vi "Problem1.9-ExecutionTime.vi"() -> ()   [LabVIEW 2019]
panel:
  out "Execution Time (ms)":dbl
  out "Min Index":i32[](array[numeric])
  out "Max Index":i32[](array[numeric])
  out "Min Value":dbl
  out "Max Value":dbl
  out "Array Size":i32[](array[numeric])
  out "Original Random Number Array":dbl[][](array[numeric])
  out "Uniform Deviates Array":dbl[][](array[numeric])
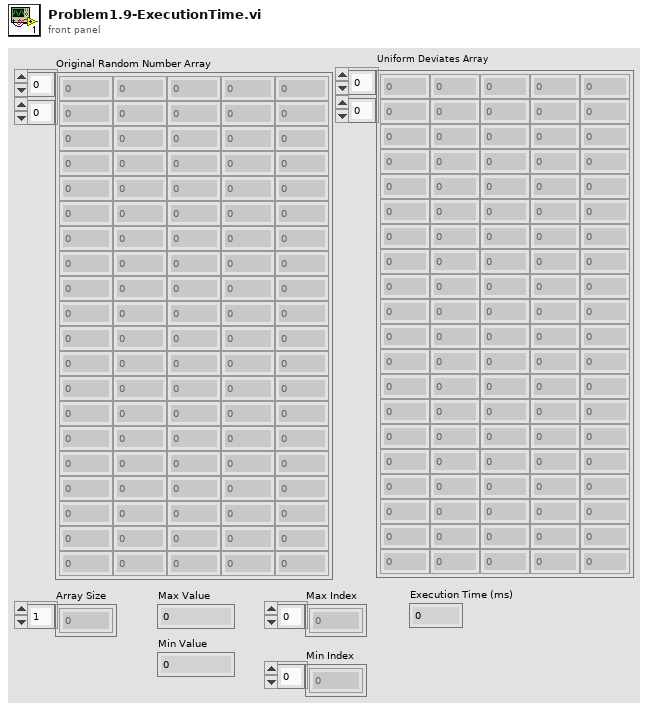
[diagram p1: front panel]
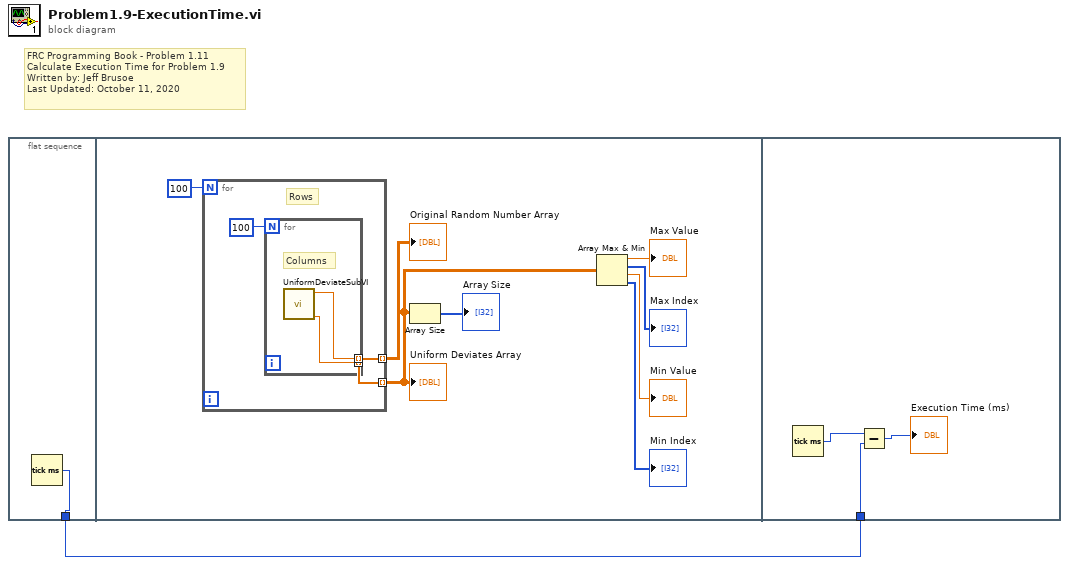
[diagram p0: block diagram]
diagram:
  # "FRC Programming Book - Problem 1.11\nCalculate Execution Time for Problem 1.9\nWritten by: Jeff Brusoe\nLast Updated: October 11, 2020"
  n1 = flat-sequence {
    tunnel: [w2] -> w1
    tunnel: w1 -> [w16]
    frame #0 {
      n2 = Tick Count (ms)() -> (millisecond timer value=w2:u32)
    }
    frame #1 {
      n3 = for {
        N: 100 -> [_]
        tunnel: [w12] -> w7 mode=indexing
        tunnel: [w11] -> w9 mode=indexing
        # "Rows"
        n4 = for {
          N: 100 -> [_]
          tunnel: [w14] -> w12 mode=indexing
          tunnel: [w15] -> w11 mode=indexing
          # "Columns"
          n5 = call "UniformDeviateSubVI.vi"() -> ("Uniform Deviate"=w14:dbl, "Initial Random Number"=w15:dbl)  [unwired: 10 in]
        }
      }
      "Uniform Deviates Array" <- w7
      "Original Random Number Array" <- w9
      n6 = Array Size(array=w7) -> (size(s)=→"Array Size":i32[])
      n7 = Array Max & Min(array=w7) -> (max value=→"Max Value":dbl, max index (indices)=→"Max Index":i32[], min value=→"Min Value":dbl, min index (indices)=→"Min Index":i32[])
    }
    frame #2 {
      n8 = Tick Count (ms)() -> (millisecond timer value=w17:u32)
      n9 = Subtract(x=w17, y=w16) -> (x-y=→"Execution Time (ms)":u32)
    }
  }
